vi "SUB_SET_DateTIME.vi"(2 "Time":string, 3 "Date":string) -> ()   [LabVIEW 2011]
panel:
  out "standard output 2":string
  out "standard output":string
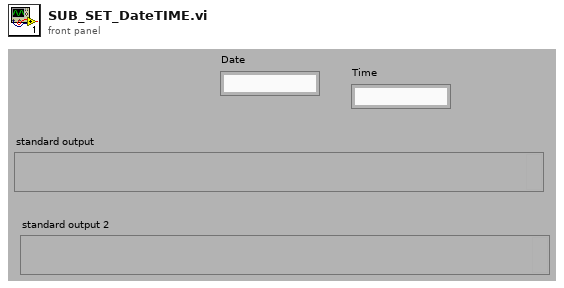
[diagram p1: front panel]
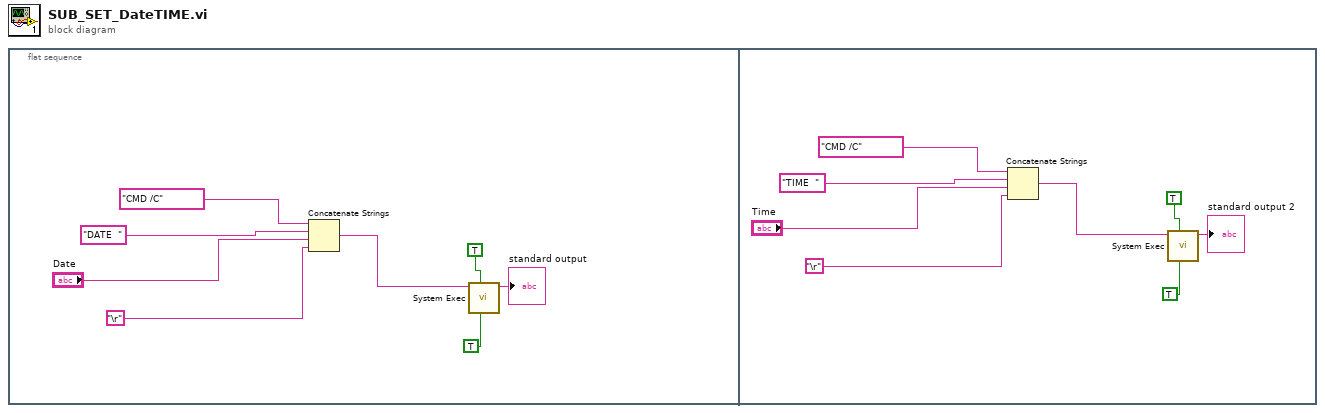
[diagram p0: block diagram]
diagram:
  n1 = flat-sequence {
    frame #0 {
      n2 = Concatenate Strings("CMD /C", "DATE  ", "Date", "\r") -> (w6:string)
      n3 = call <vilib>:"System Exec.vi"("run minimized? (F)"=TRUE, "wait until completion? (T)"=TRUE, "command line"=w6) -> ("standard output"=→"standard output":string)  [unwired: 5 in, 3 out]
    }
    frame #1 {
      n4 = Concatenate Strings("CMD /C", "TIME  ", "Time", "\r") -> (w14:string)
      n5 = call <vilib>:"System Exec.vi"("run minimized? (F)"=TRUE, "wait until completion? (T)"=TRUE, "command line"=w14) -> ("standard output"=→"standard output 2":string)  [unwired: 5 in, 3 out]
    }
  }
